vi "Start_stop_calculations.vi"(3 "Binary SICK":i16[](array[numeric])) -> (0 "Number of Valleys":i16, 1 "Stop":i16[](array[numeric]), 2 "Start":i16[](array[numeric]))   [LabVIEW 2009]
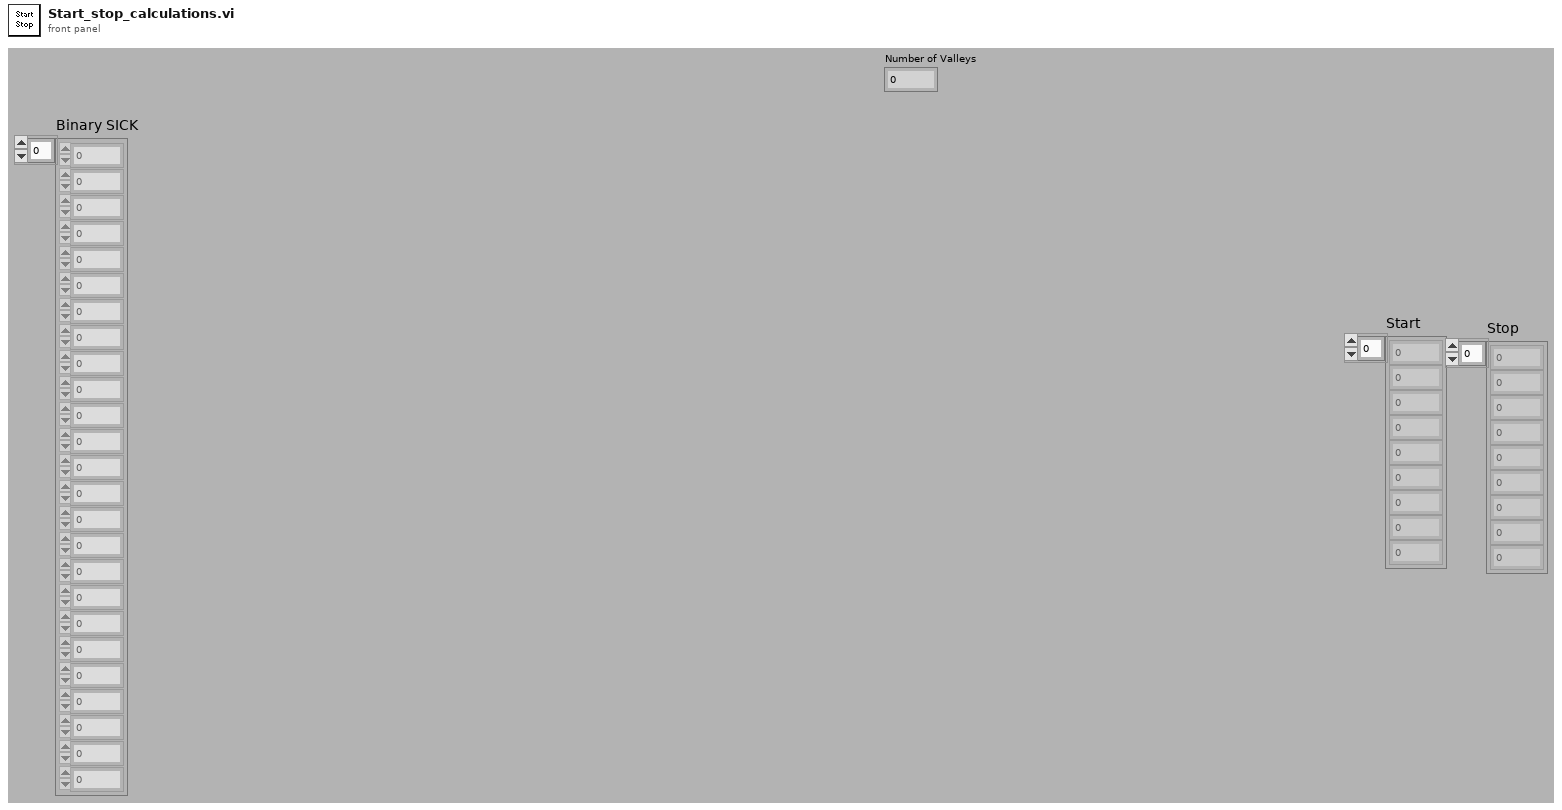
[diagram p1: front panel]
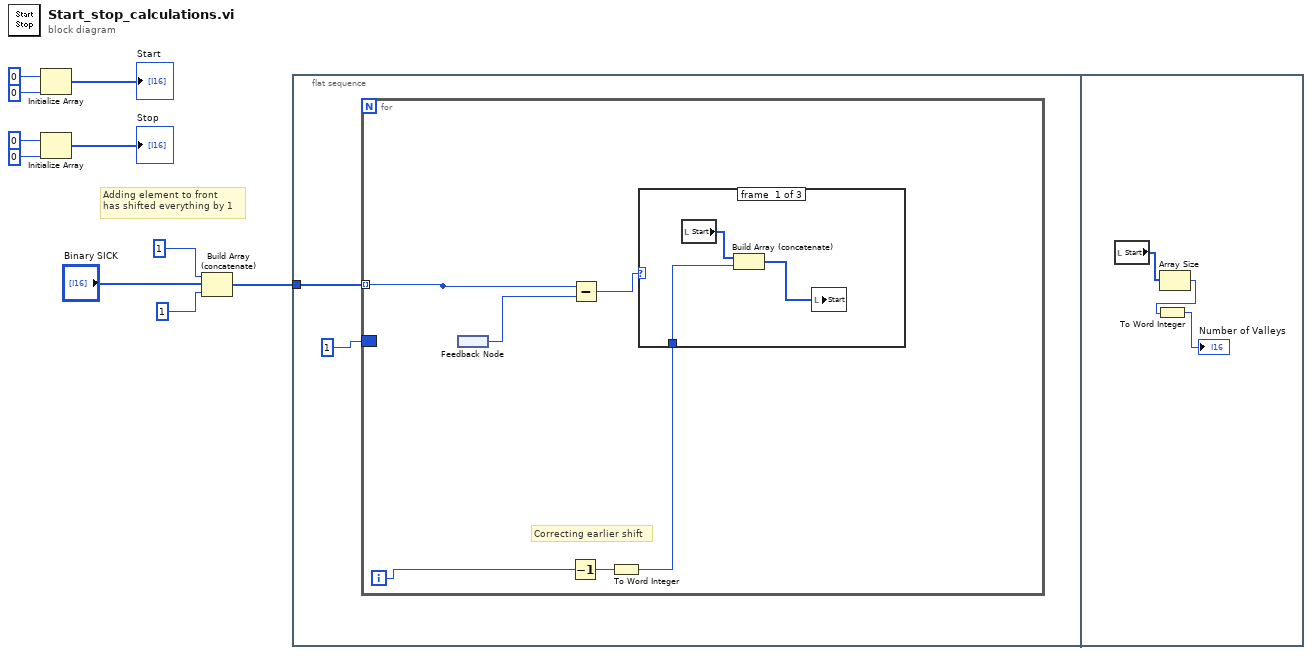
[diagram p0: block diagram]
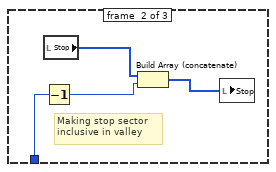
[diagram p2: hidden frame]
diagram:
  # "Adding element to front\nhas shifted everything by 1"
  n1 = Initialize Array(i16 0 ("element"), 0 ("dimension size")) -> (→"Start":i16[])
  n2 = Initialize Array(i16 0 ("element"), 0 ("dimension size")) -> (→"Stop":i16[])
  n3 = Build Array (concatenate)(i16 1, "Binary SICK", i16 1) -> (w6:i16[])
  n4 = flat-sequence {
    tunnel: w6 -> [w12]
    frame #0 {
      n5 = for {
        tunnel: w12 -> [w17] mode=indexing
        border: i16 1 -> [_]
        i -> [w16]
        # "Correcting earlier shift"
        n6 = feedback #1() -> (w13:i16)
        n7 = Decrement(x=w16) -> (x-1=w15:i32)
        n8 = Subtract(x=w17, y=w13) -> (x-y=w18:i16)
        n9 = To Word Integer(number=w15) -> (16bit integer=w14:i16)
        n10 = case shown="1" w18 {
          tunnel: w14 -> [w21 w22 _]
          frame #0 {
            n11 = local read "Start"() -> (w19:i16[])
            n12 = Build Array (concatenate)(w19, w21) -> (w20:i16[])
            n13 = local write "Start"(w20) -> ()
          }
          frame #1 {
            # "Making stop sector \ninclusive in valley"
            n14 = local read "Stop"() -> (w24:i16[])
            n15 = Decrement(x=w22) -> (x-1=w23:i16)
            n16 = Build Array (concatenate)(w24, w23) -> (w25:i16[])
            n17 = local write "Stop"(w25) -> ()
          }
          frame #2 {
          }
        }
      }
    }
    frame #1 {
      n18 = local read "Start"() -> (w28:i16[])
      n19 = Array Size(array=w28) -> (size(s)=w27:i32)
      n20 = To Word Integer(number=w27) -> (16bit integer=→"Number of Valleys":i16)
    }
  }
